vi "Get Test by GUID.vi"(8 "error in":errorcluster, 10 "GUID":string, 11 "AllTests":refnum<class>[](array[class])) -> (0 "error out":errorcluster, 1 "Found":bool, 2 "Test":refnum<class>)   [LabVIEW 2011, in "GraphicalTestRunner.lvlib"]
uses:
  GraphicalTestRunner.lvlib
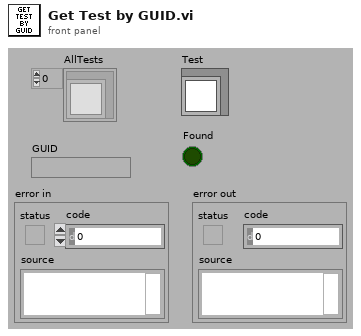
[diagram p1: front panel]
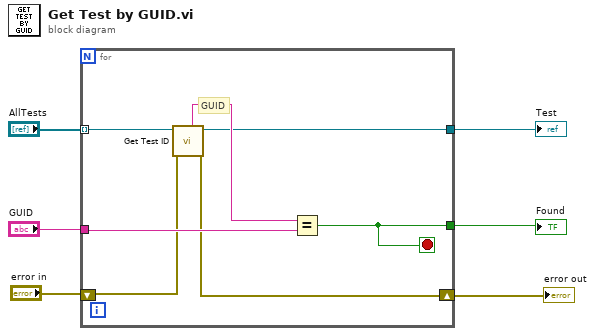
[diagram p0: block diagram]
diagram:
  n1 = for {
    tunnel: "AllTests" -> [w10] mode=indexing
    tunnel: "GUID" -> [w13]
    tunnel: [w9] -> w6
    tunnel: [w12] -> w3
    shift-right: [w7] -> w1
    shift-left: "error in" -> [w8]
    stop <- w12 stop-if-true
    # "GUID"
    n2 = call "Get Test ID.vi"("error in"=w8, "Test In"=w10) -> ("error out"=w7:errorcluster, "Test Out"=w9:refnum<class>, "GUID"=w11:string)  [unwired: 5 in, 2 out]
    n3 = Equal?(x=w11, y=w13) -> (x = y?=w12:bool)
  }
  "Test" <- w6
  "Found" <- w3
  "error out" <- w1
